vi "ABS Pos Cal.vi"(8 "error in (no error)":errorcluster, 9 "Init Pul Num":i32, 10 "Data":u8[](array[numeric]), 11 "SGDV_Ctrl_Class in":refnum<class "SGDV_Ctrl_Class.lvclass">) -> (0 "error out":errorcluster, 1 "Get Serial Data?":bool, 2 "Init-Enc-Pos (cnt)":dbl, 3 "SGDV_Ctrl_Class out":refnum<class "SGDV_Ctrl_Class.lvclass">, 4 "Init Motor Data":T1)   [LabVIEW 2013, in "SGDV_Ctrl_v13_lib.lvlib" / "SGDV_Ctrl_Class.lvclass"]
uses:
  SGDV_Ctrl_Class.lvclass
  Controls and General VIs/Init Motor Data.ctl
  SGDV_Ctrl_Class.lvclass/SGDV_Ctrl_Class.ctl
  SGDV_Ctrl_v13_lib.lvlib
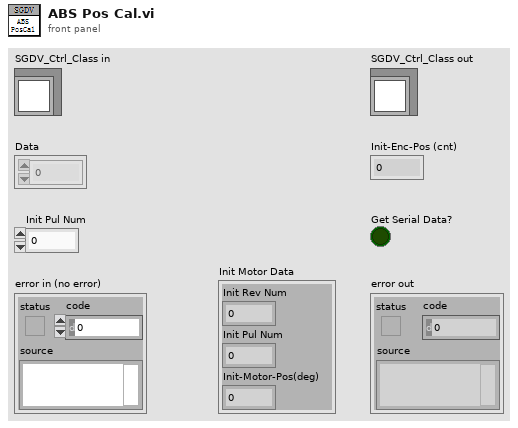
[diagram p1: front panel]
types:
  T1 = typedef "SGDV_Ctrl_v13_lib.lvlib/Init Motor Data.ctl" = cluster{"Init Rev Num":i32, "Init Pul Num":i32, "Init-Motor-Pos(deg)":dbl}
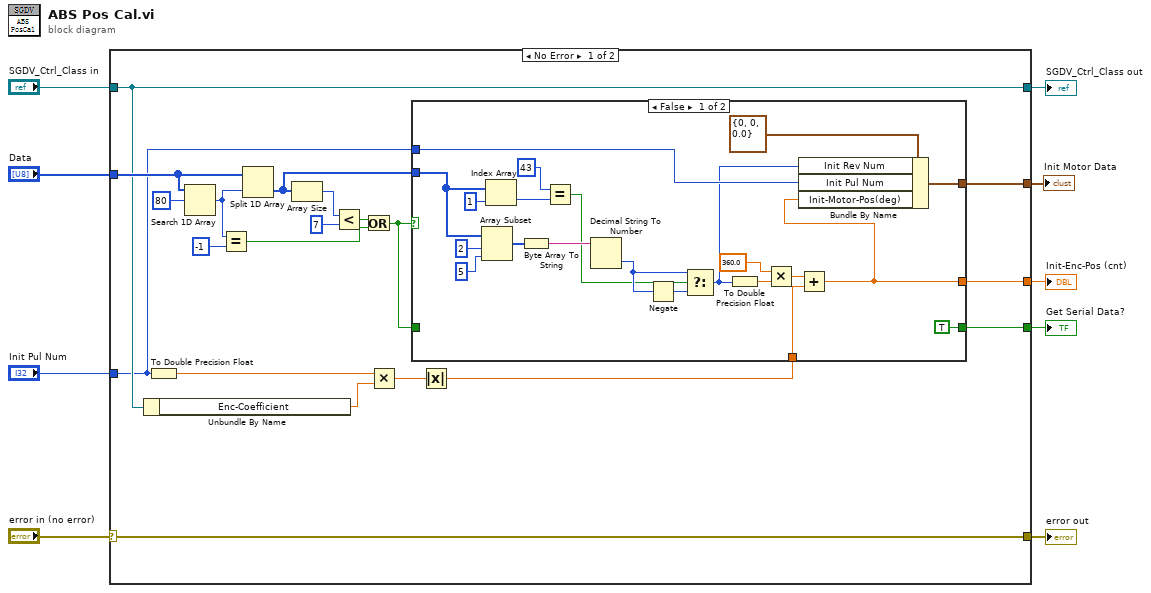
[diagram p0: block diagram]
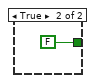
[diagram p2: hidden frame]
diagram:
  n1 = case shown="No Error" "error in (no error)" {
    selector: "error in (no error)" -> [w29 w53]
    tunnel: [w29 w53] -> w2
    tunnel: [w18 w52] -> w5
    tunnel: "SGDV_Ctrl_Class in" -> [w18 w52]
    tunnel: "Data" -> [w27 _]
    tunnel: [w19 _] -> w4
    tunnel: [w16 _] -> w3
    tunnel: "Init Pul Num" -> [w11 _]
    tunnel: [w10 _] -> w1
    frame No Error {
      n2 = Unbundle By Name(w18) -> ("Enc-Coefficient"=w15:dbl)
      n3 = To Double Precision Float(number=w11) -> (double precision float=w13:dbl)
      n4 = Search 1D Array(1D array=w27, element=u8 80 ("x")) -> (index of element=w25:i32)  [unwired: 1 in]
      n5 = Equal?(x=w25, y=-1) -> (x = y?=w21:bool)
      n6 = Split 1D Array(array=w27, index=w25) -> (second subarray=w20:u8[])  [unwired: 1 out]
      n7 = Array Size(array=w20) -> (size(s)=w24:i32)
      n8 = Less?(x=w24, y=7) -> (x < y?=w22:bool)
      n9 = Or(x=w22, y=w21) -> (x .or. y?=w17:bool)
      n10 = Multiply(x=w13, y=w15) -> (x*y=w14:dbl)
      n11 = Absolute Value(x=w14) -> (abs(x)=w12:dbl)
      n12 = case shown="False" w17 {
        tunnel: w20 -> [w40 _]
        tunnel: [w30 _] -> w19
        tunnel: w17 -> [_ _]
        tunnel: [TRUE FALSE] -> w16
        tunnel: w12 -> [w37 _]
        tunnel: w11 -> [w35 _]
        tunnel: [w34 _] -> w10
        frame False {
          n13 = Array Subset(array=w40, index=2, length=5) -> (w41:u8[])
          n14 = Index Array(array=w40, index=1) -> (element=w45:u8)
          n15 = Byte Array To String(unsigned byte array=w41) -> (string=w47:string)
          n16 = Equal?(x=u8 43, y=w45) -> (x = y?=w39:bool)
          n17 = Decimal String To Number(string=w47) -> (number=w43:i32)  [unwired: 2 in, 1 out]
          n18 = Negate(x=w43) -> (-x=w42:i32)
          n19 = Select(t=w43, s=w39, f=w42) -> (s? t:f=w32:i32)
          n20 = To Double Precision Float(number=w32) -> (double precision float=w31:dbl)
          n21 = Multiply(x=360.0, y=w31) -> (x*y=w38:dbl)
          n22 = Add(x=w38, y=w37) -> (x+y=w30:dbl)
          n23 = Bundle By Name(cluster=T1 {"Init Rev Num"=0, "Init Pul Num"=0, "Init-Motor-Pos(deg)"=0.0} ("Init Motor Data"), "Init Rev Num"=w32, "Init Pul Num"=w35, "Init-Motor-Pos(deg)"=w30) -> (w34:T1)
        }
        frame True {
        }
      }
    }
    frame Error {
    }
  }
  "error out" <- w2
  "SGDV_Ctrl_Class out" <- w5
  "Init-Enc-Pos (cnt)" <- w4
  "Get Serial Data?" <- w3
  "Init Motor Data" <- w1
